vi "ln(x).vi"(1 "x":fxp<+,8,0>) -> (0 "ln(x)":fxp<+/-,33,4>)   [LabVIEW 2020]
uses:
  <vilib>/rvi/FXPMathLib/FxpLn/subVIs/nifxpmath_NaturalLogarithm_SimConfig.ctl
  <vilib>/rvi/FXPMathLib/FxpLn/simVIs/DllFxpNaturalLogarithmTemp_sub.vi
  <vilib>/rvi/FXPMathLib/FxpInterpret/XNode/nifxpmath_Interpret.xnode
  <vilib>/rvi/FXPMathLib/FxpLn/XNode/nifxpmath_NaturalLogarithm.xnode
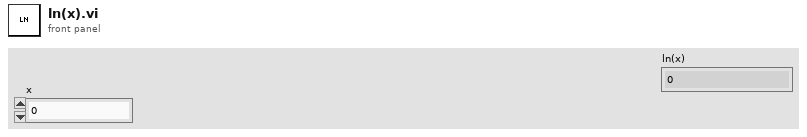
[diagram p1: front panel]
types:
  T1 = enum8{"128", "64", "32", "16", "8", "4", "2", "1"}
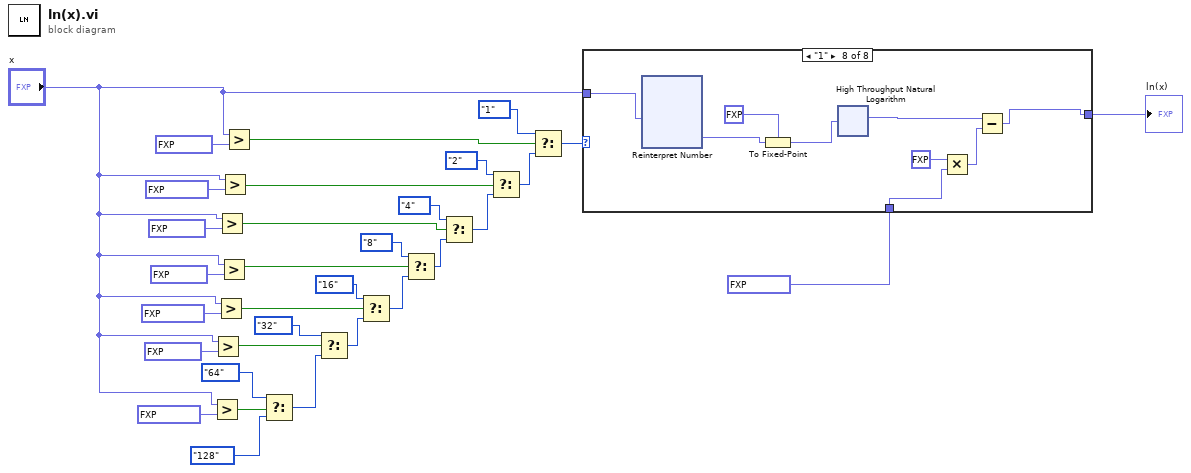
[diagram p0: block diagram]
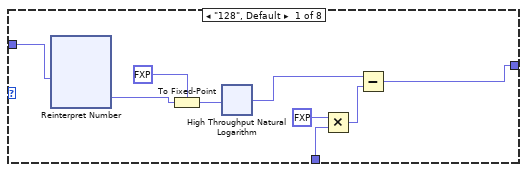
[diagram p2: hidden frame]
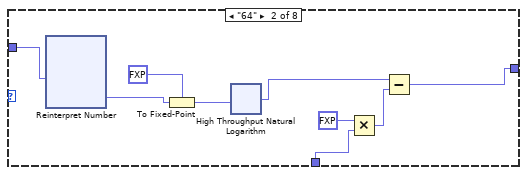
[diagram p3: hidden frame]
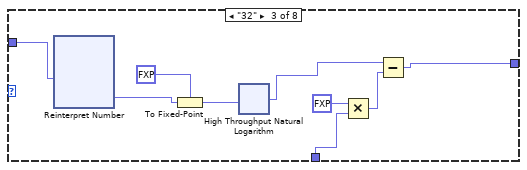
[diagram p4: hidden frame]
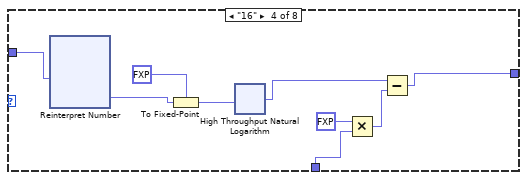
[diagram p5: hidden frame]
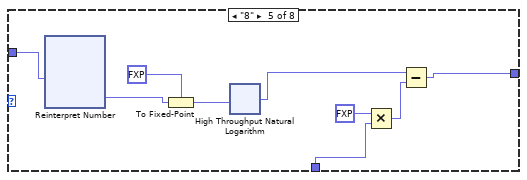
[diagram p6: hidden frame]
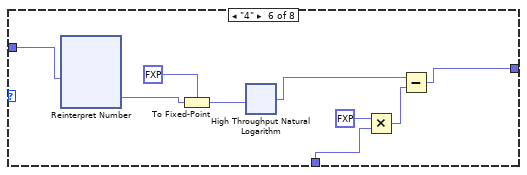
[diagram p7: hidden frame]
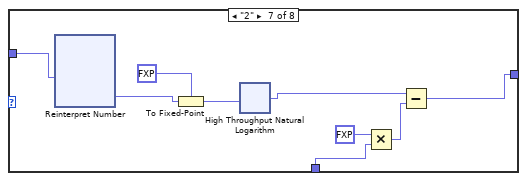
[diagram p8: hidden frame]
diagram:
  n1 = Greater?(x="x", y=fxp<+,8,0> 0.00390625) -> (0:w24:bool)
  n2 = Greater?(x="x", y=fxp<+,8,0> 0.0078125) -> (0:w6:bool)
  n3 = Greater?(x="x", y=fxp<+,8,0> 0.01953125) -> (0:w10:bool)
  n4 = Greater?(x="x", y=fxp<+,8,0> 0.0859375) -> (0:w16:bool)
  n5 = Greater?(x="x", y=fxp<+,8,0> 0.4296875) -> (0:w13:bool)
  n6 = Greater?(x="x", y=fxp<+,8,0> 0.18359375) -> (0:w22:bool)
  n7 = Greater?(x="x", y=fxp<+,8,0> 0.3671875) -> (0:w31:bool)
  n8 = Select(t=T1."64", s=w24, f=T1."128") -> (s? t:f=w4:T1)
  n9 = Select(t=T1."32", s=w6, f=w4) -> (s? t:f=w7:T1)
  n10 = Select(t=T1."16", s=w10, f=w7) -> (s? t:f=w11:T1)
  n11 = Select(t=T1."8", s=w13, f=w11) -> (s? t:f=w14:T1)
  n12 = Select(t=T1."4", s=w16, f=w14) -> (s? t:f=w17:T1)
  n13 = Select(t=T1."2", s=w22, f=w17) -> (s? t:f=w20:T1)
  n14 = Select(t=T1."1", s=w31, f=w20) -> (s? t:f=w19:T1)
  n15 = case shown="\"1\"" w19 {
    tunnel: [w33 w67 w101 w136 w169 w203 w237 w275] -> w1
    tunnel: "x" -> [w38 w72 w106 w140 w174 w208 w245 w272]
    tunnel: fxp<+,8,0> 0.69140625 ("y") -> [w37 w68 w103 w135 w170 w205 w239 w277]
    frame "128", Default {
      n16 = xnode "Reinterpret Number"("x"=w38) -> ("y"=w39:fxp<+,8,7>)
      n17 = To Fixed-Point(fixed-point type=fxp<+,8,0> 0.0 ("y"), number=w39) -> (fixed-point=w41:fxp<+,8,0>)
      n18 = xnode "High Throughput Natural Logarithm"("x"=w41) -> ("ln(x)"=w34:fxp<+/-,30,1>)  [unwired: 1 out]
      n19 = Multiply(x=fxp<+,3,3> 7.0, y=w37) -> (x*y=w35:fxp<+,11,3>)
      n20 = Subtract(x=w34, y=w35) -> (x-y=w33:fxp<+/-,33,4>)
    }
    frame "64" {
      n21 = xnode "Reinterpret Number"("x"=w72) -> ("y"=w73:fxp<+,8,6>)
      n22 = To Fixed-Point(fixed-point type=fxp<+,8,0> 0.0 ("y"), number=w73) -> (fixed-point=w75:fxp<+,8,0>)
      n23 = xnode "High Throughput Natural Logarithm"("x"=w75) -> ("ln(x)"=w69:fxp<+/-,30,1>)  [unwired: 1 out]
      n24 = Multiply(x=fxp<+,3,3> 6.0, y=w68) -> (x*y=w70:fxp<+,11,3>)
      n25 = Subtract(x=w69, y=w70) -> (x-y=w67:fxp<+/-,33,4>)
    }
    frame "32" {
      n26 = xnode "Reinterpret Number"("x"=w106) -> ("y"=w107:fxp<+,8,5>)
      n27 = To Fixed-Point(fixed-point type=fxp<+,8,0> 0.0 ("y"), number=w107) -> (fixed-point=w109:fxp<+,8,0>)
      n28 = xnode "High Throughput Natural Logarithm"("x"=w109) -> ("ln(x)"=w102:fxp<+/-,30,1>)  [unwired: 1 out]
      n29 = Multiply(x=fxp<+,3,3> 5.0, y=w103) -> (x*y=w104:fxp<+,11,3>)
      n30 = Subtract(x=w102, y=w104) -> (x-y=w101:fxp<+/-,33,4>)
    }
    frame "16" {
      n31 = xnode "Reinterpret Number"("x"=w140) -> ("y"=w141:fxp<+,8,4>)
      n32 = To Fixed-Point(fixed-point type=fxp<+,8,0> 0.0 ("y"), number=w141) -> (fixed-point=w143:fxp<+,8,0>)
      n33 = xnode "High Throughput Natural Logarithm"("x"=w143) -> ("ln(x)"=w137:fxp<+/-,30,1>)  [unwired: 1 out]
      n34 = Multiply(x=fxp<+,3,3> 4.0, y=w135) -> (x*y=w138:fxp<+,11,3>)
      n35 = Subtract(x=w137, y=w138) -> (x-y=w136:fxp<+/-,33,4>)
    }
    frame "8" {
      n36 = xnode "Reinterpret Number"("x"=w174) -> ("y"=w175:fxp<+,8,3>)
      n37 = To Fixed-Point(fixed-point type=fxp<+,8,0> 0.0 ("y"), number=w175) -> (fixed-point=w177:fxp<+,8,0>)
      n38 = xnode "High Throughput Natural Logarithm"("x"=w177) -> ("ln(x)"=w171:fxp<+/-,30,1>)  [unwired: 1 out]
      n39 = Multiply(x=fxp<+,3,3> 3.0, y=w170) -> (x*y=w172:fxp<+,11,3>)
      n40 = Subtract(x=w171, y=w172) -> (x-y=w169:fxp<+/-,33,4>)
    }
    frame "4" {
      n41 = xnode "Reinterpret Number"("x"=w208) -> ("y"=w209:fxp<+,8,2>)
      n42 = To Fixed-Point(fixed-point type=fxp<+,8,0> 0.0 ("y"), number=w209) -> (fixed-point=w211:fxp<+,8,0>)
      n43 = xnode "High Throughput Natural Logarithm"("x"=w211) -> ("ln(x)"=w204:fxp<+/-,30,1>)  [unwired: 1 out]
      n44 = Multiply(x=fxp<+,3,3> 2.0, y=w205) -> (x*y=w206:fxp<+,11,3>)
      n45 = Subtract(x=w204, y=w206) -> (x-y=w203:fxp<+/-,33,4>)
    }
    frame "2" {
      n46 = xnode "Reinterpret Number"("x"=w245) -> ("y"=w242:fxp<+,8,1>)
      n47 = To Fixed-Point(fixed-point type=fxp<+,8,0> 0.0 ("y"), number=w242) -> (fixed-point=w244:fxp<+,8,0>)
      n48 = xnode "High Throughput Natural Logarithm"("x"=w244) -> ("ln(x)"=w238:fxp<+/-,30,1>)  [unwired: 1 out]
      n49 = Multiply(x=fxp<+,3,3> 1.0, y=w239) -> (x*y=w240:fxp<+,11,3>)
      n50 = Subtract(x=w238, y=w240) -> (x-y=w237:fxp<+/-,33,4>)
    }
    frame "1" {
      n51 = xnode "Reinterpret Number"("x"=w272) -> ("y"=w273:fxp<+,8,0>)
      n52 = To Fixed-Point(fixed-point type=fxp<+,8,0> 0.0 ("y"), number=w273) -> (fixed-point=w271:fxp<+,8,0>)
      n53 = xnode "High Throughput Natural Logarithm"("x"=w271) -> ("ln(x)"=w276:fxp<+/-,30,1>)  [unwired: 1 out]
      n54 = Multiply(x=fxp<+,3,3> 0.0, y=w277) -> (x*y=w278:fxp<+,11,3>)
      n55 = Subtract(x=w276, y=w278) -> (x-y=w275:fxp<+/-,33,4>)
    }
  }
  "ln(x)" <- w1
